vi "Arduino End Comms.vi"(1 "Resource index":i32) -> (0 "Error":errorcluster, 2 "Arduino VISA config & resource":T1={"VISA resource name"="COM12", "baud rate (bps)"=276000, "timeout (ms)"=12000, "data bits"=8, "parity"=enum."None", "stop bits (10: 1 bit)"=10, "flow control"=0, "termination char (hex)"=10, "Enable Termination Char"=FALSE, "byte count"=12, "Resource locked?"=FALSE} {"termination char (hex)" format="%02x"; "stop bits (10: 1 bit)" items=["1.0"=10, "1.5"=15, "2.0"=20]; "flow control" items=["None", "XON/XOFF", "RTS/CTS", "XON/XOFF & RTS/CTS", "DTR/DSR", "XON/XOFF & DTR/DSR"]})   [LabVIEW 2013]
uses:
  ctls_and_globals/Arduino Config & resource typedef.ctl
  ctls_and_globals/Arduino Global.vi
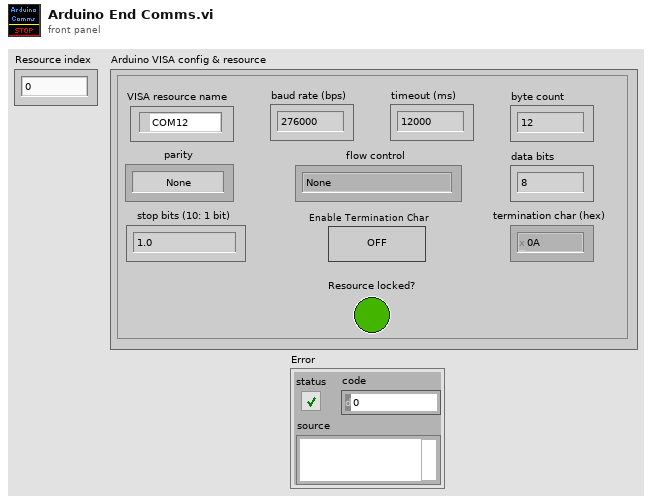
[diagram p1: front panel]
types:
  T1 = typedef "Arduino Config & resource typedef.ctl" = cluster{"VISA resource name":refnum<visa-resource-name>, "baud rate (bps)":u32, "timeout (ms)":u32, "data bits":u16, "parity":enum16{"None", "Odd", "Even", "Mark", "Space"}, "stop bits (10: 1 bit)":u16, "flow control":u16, "termination char (hex)":u8, "Enable Termination Char":bool, "byte count":u32, "Resource locked?":bool}
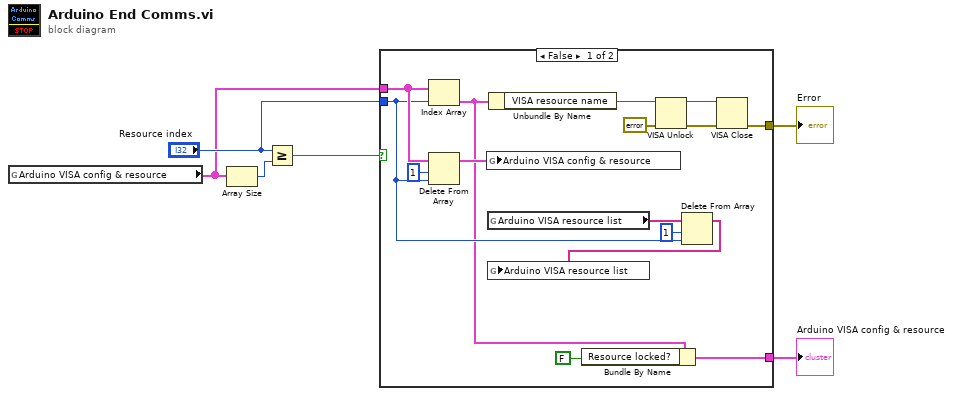
[diagram p0: block diagram]
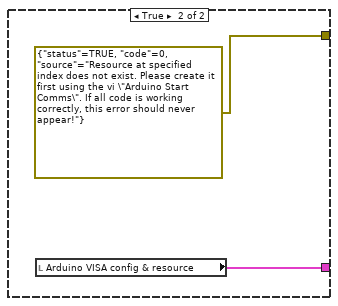
[diagram p2: hidden frame]
diagram:
  n1 = global read "Arduino Global.vi" "Arduino VISA config & resource"() -> (w2:T1[])
  n2 = Array Size(array=w2) -> (size(s)=w6:i32)
  n3 = Greater Or Equal?(x="Resource index", y=w6) -> (x >= y?=w5:bool)
  n4 = case shown="False" w5 {
    tunnel: [w17 errorcluster {"status"=TRUE, "code"=0, "source"="Resource at specified index does not exist. Please create it first using the vi \"Arduino Start Comms\". If all code is working correctly, this error should never appear!"} ("error out")] -> w4
    tunnel: "Resource index" -> [w9 _]
    tunnel: w2 -> [w16 _]
    tunnel: [w12 w22] -> w1
    frame False {
      n5 = Index Array(array=w16, index=w9) -> (element=w7:T1)
      n6 = Delete From Array(array=w16, length=1, index=w9) -> (array with subset deleted=w14:T1[])  [unwired: 1 out]
      n7 = global write "Arduino Global.vi" "Arduino VISA config & resource"(w14) -> ()
      n8 = global read "Arduino Global.vi" "Arduino VISA resource list"() -> (w10:string[])
      n9 = Unbundle By Name(w7) -> ("VISA resource name"=w19:refnum<visa-resource-name>)
      n10 = Bundle By Name(cluster=w7, "Resource locked?"=FALSE) -> (w12:T1)
      n11 = VISA Unlock(8:errorcluster {"status"=FALSE, "code"=0, "source"=""} ("error in (no error)"), 11:w19) -> (0:w20:errorcluster, 3:w21:refnum<visa-resource-name>)
      n12 = Delete From Array(array=w10, length=1, index=w9) -> (array with subset deleted=w8:string[])  [unwired: 1 out]
      n13 = global write "Arduino Global.vi" "Arduino VISA resource list"(w8) -> ()
      n14 = VISA Close(VISA resource name=w21, error in (no error)=w20) -> (error out=w17:errorcluster)
    }
    frame True {
      n15 = local read "Arduino VISA config & resource"() -> (w22:T1)
    }
  }
  "Arduino VISA config & resource" <- w1
  "Error" <- w4
